vi "_propertyNode.vi"   [LabVIEW 2013, in "BSON.lvlib"]
uses:
  BSON.lvlib
  tBSONDocument.lvclass
  getElements.vi
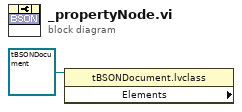
[diagram p0: block diagram]
diagram:
  n1 = property class="tBSONDocument.lvclass" props=["Elements"](reference=refnum<class "tBSONDocument.lvclass"> refnum) -> ()  [unwired: 1 in, 3 out]
